vi "TRITON_TEMP_SPEC.vi"(1 "Target Temperature [K]":dbl) -> (0 "Temperature Stability Specification":dbl)   [LabVIEW 2009]
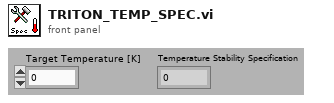
[diagram p1: front panel]
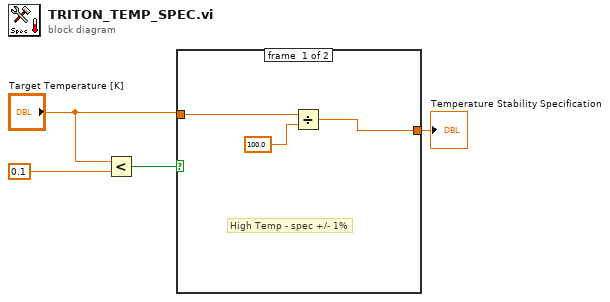
[diagram p0: block diagram]
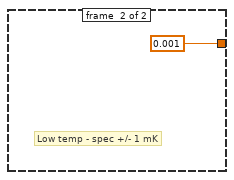
[diagram p2: hidden frame]
diagram:
  n1 = Less?(x="Target Temperature [K]", y=0.1) -> (x < y?=w3:bool)
  n2 = case shown="True" w3 {
    tunnel: "Target Temperature [K]" -> [w7 _]
    tunnel: [w5 0.001] -> w1
    frame #0 {
      # "High Temp - spec +/- 1%"
      n3 = Divide(x=w7, y=100.0) -> (x/y=w5:dbl)
    }
    frame #1 {
      # "Low temp - spec +/- 1 mK"
    }
  }
  "Temperature Stability Specification" <- w1
